vi "clearpath_parse_power_status.vi"(0 "ClearpathComm":T1) -> (1 "Data Valid?":bool=TRUE, 2 "Capacity":i16, 3 "Flags":u8 format="%b", 4 "Charge":dbl)   [LabVIEW 2010, in "clearpath_interface.lvlib"]
doc: "Parses current status of platform power system. (Message type 0x8005)"
uses:
  clearpath_interface.lvlib
  cwrap_cRIO.dll
panel:
  # "Power System Status"
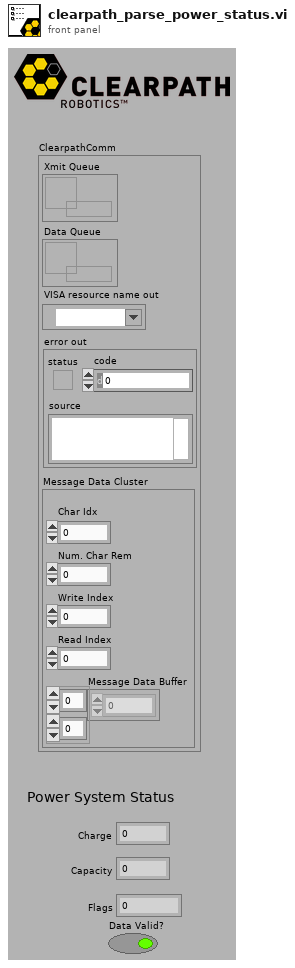
[diagram p1: front panel]
types:
  T1 = cluster{"Xmit Queue":refnum<queue>, "Data Queue":refnum<queue>, "VISA resource name out":refnum<visa-resource-name>, "error out":errorcluster, "Message Data Cluster":cluster{"\nChar Idx":u8, "Num. Char Rem":u8, "Write Index":u8, "Read Index":u8, "Message Data Buffer":u8[][]}}
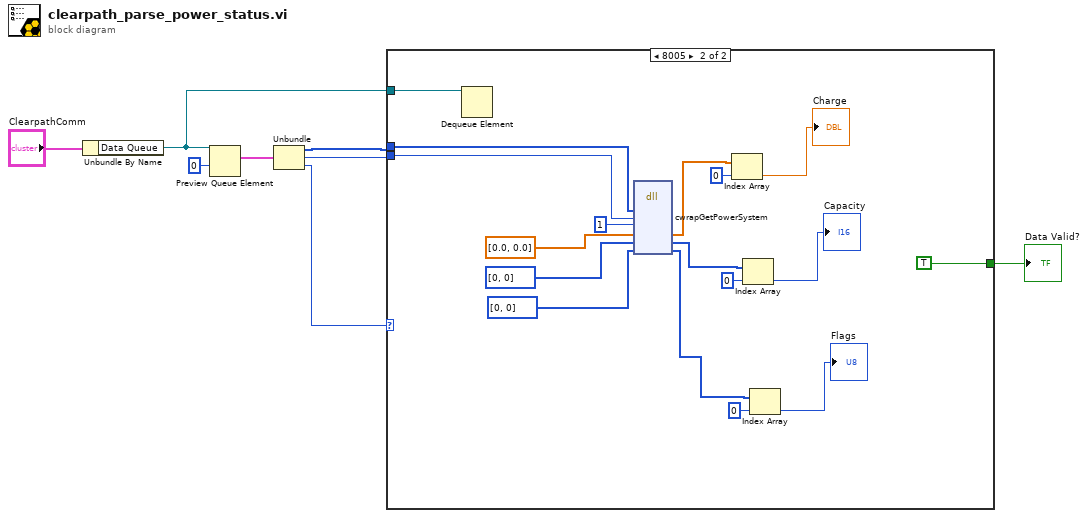
[diagram p0: block diagram]
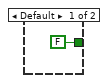
[diagram p2: hidden frame]
diagram:
  n1 = Unbundle By Name("ClearpathComm") -> ("Data Queue"=w1:refnum<queue>)
  n2 = Preview Queue Element(queue=w1, timeout in ms (-1)=0) -> (element=w6:cluster{u8[], "Length":i32, "Type":i32})  [unwired: 1 in, 3 out]
  n3 = Unbundle(w6) -> (w3:u8[], "Length"=w4:i32, "Type"=w5:i32)
  n4 = case shown="8005" w5 {
    tunnel: w4 -> [_ w12]
    tunnel: w3 -> [_ w13]
    tunnel: [FALSE TRUE] -> w2
    tunnel: w1 -> [_ w10]
    frame Default {
    }
    frame 32773 {
      n5 = Dequeue Element(queue=w10) -> ()  [unwired: 2 in, 4 out]
      n6 = dll-call lib="cwrap_cRIO.*" fn="cwrapGetPowerSystem"("packet"=w13, "len"=w12, "bat_count"=i8 1 ("enc_count"), "charge_est"=dbl[] [0.0, 0.0] ("Array"), "cap_est"=i16[] [0, 0] ("Array"), "desc"=u8[] [0, 0] ("Array")) -> ("charge_est"=w20:dbl[], "cap_est"=w14:i16[], "desc"=w15:u8[])  [unwired: 7 in, 2 out]
      n7 = Index Array(array=w20, index=0) -> (element=→"Charge":dbl)
      n8 = Index Array(array=w14, index=0) -> (element=→"Capacity":i16)
      n9 = Index Array(array=w15, index=0) -> (element=→"Flags":u8)
    }
  }
  "Data Valid?" <- w2
